vi "ADIS16470 Reset.vi"(8 "error in (no error)":errorcluster, 10 "Reset?":bool, 11 "ADIS16470DevRef":T1) -> (0 "error out":errorcluster, 3 "ADIS16470DevRef":T1)   [LabVIEW 2018]
uses:
  Typedef/ADIS16470 Device Reference.ctl
  Typedef/ADIS16470 Hardware Configuration.ctl
  <vilib>/Rock Robotics/WPI/SPI/WPI_SPIMode.ctl
  <vilib>/Rock Robotics/SystemInterfaces/DIO/FPGA_DIOChannel.ctl
  <vilib>/Rock Robotics/SystemInterfaces/spilib/spi_bus.ctl
  Typedef/ADIS16470 Data.ctl
  Typedef/ADIS16470 Status.ctl
  Typedef/ADIS16470 Process.ctl
  Typedef/ADIS16470 Command Type.ctl
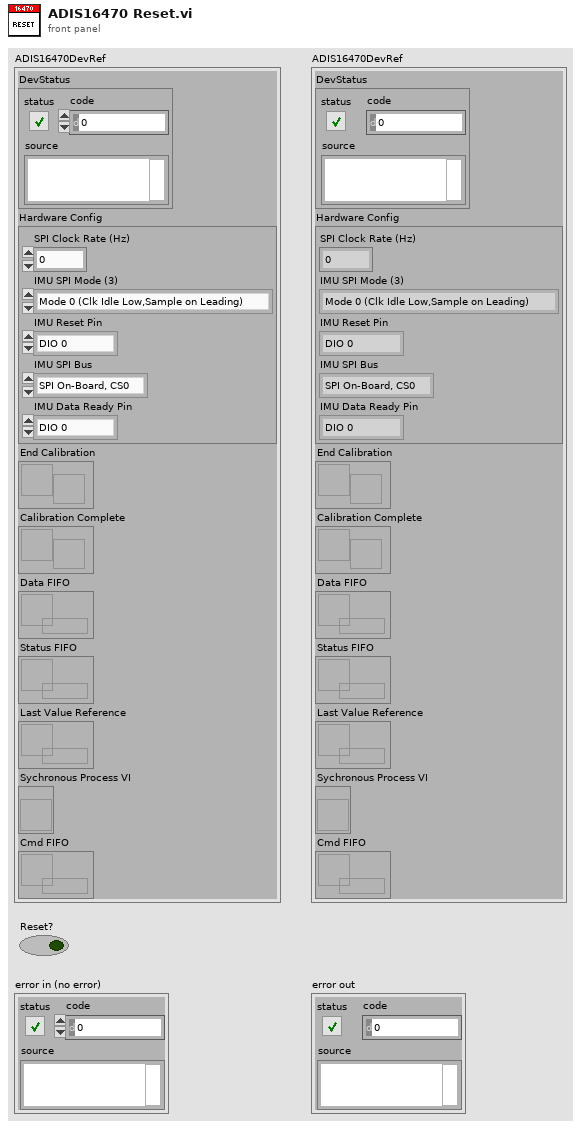
[diagram p1: front panel]
types:
  T1 = typedef "ADIS16470 Device Reference.ctl" = cluster{"DevStatus":errorcluster, "Hardware Config":T2, "End Calibration":refnum<notifier>, "Calibration Complete":refnum<notifier>, "Data FIFO":refnum<k33>, "Status FIFO":refnum<k33>, "Last Value Reference":refnum<data-value>, "Sychronous Process VI":T6, "Cmd FIFO":refnum<k33>}
  T2 = typedef "ADIS16470 Hardware Configuration.ctl" = cluster{"SPI Clock Rate (Hz)":dbl, "IMU SPI Mode (3)":T3, "IMU Reset Pin":T4, "IMU SPI Bus":T5, "IMU Data Ready Pin":T4}
  T3 = typedef "WPI_SPIMode.ctl" = enum16{"Mode 0 (Clk Idle Low,Sample on Leading)", "Mode 1 (Clk Idle Low,Sample on Trailing)", "Mode 2 (Clk Idle High,Sample on Leading)", "Mode 3 (Clk Idle High,Sample on Trailing)"}
  T4 = typedef "FPGA_DIOChannel.ctl" = enum8{"DIO 0", "DIO 1", "DIO 2", "DIO 3", "DIO 4", "DIO 5", "DIO 6", "DIO 7", "DIO 8", "DIO 9", "DIO MXP 0", "DIO MXP 1", "DIO MXP 2", "DIO MXP 3", "DIO MXP 4", "DIO MXP 5", "DIO MXP 6", "DIO MXP 7", "DIO MXP 8", "DIO MXP 9", "DIO MXP 10", "DIO MXP 11", "DIO MXP 12", "DIO MXP 13", "DIO MXP 14", "DIO MXP 15", "SPI Port CS1", "SPI Port CS2", "SPI Port CS3", "SPI Port MISO", "SPI Port MOSI", "Invalid"}
  T5 = typedef "spi_bus.ctl" = enum16{"SPI On-Board, CS0", "SPI On-Board, CS1", "SPI On-Board, CS2", "SPI On-Board, CS3", "SPI MXP", "Invalid"}
  T6 = typedef "ADIS16470 Process.ctl" = refnum<vi>
  T7 = typedef "ADIS16470 Command Type.ctl" = enum16{"None", "Reset"}
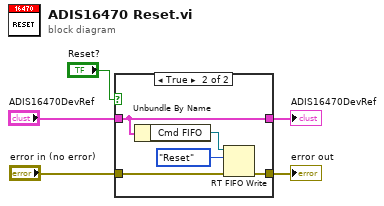
[diagram p0: block diagram]
diagram:
  n1 = case shown="True" "Reset?" {
    tunnel: "ADIS16470DevRef" -> [w6 w10]
    tunnel: "error in (no error)" -> [w7 w12]
    tunnel: [w7 w11] -> w4
    tunnel: [w6 w10] -> w5
    frame False {
    }
    frame True {
      n2 = Unbundle By Name(w10) -> ("Cmd FIFO"=w9:refnum<k33>)
      n3 = RT FIFO Write(0:w9, 1:ADIS16470_Command_Type."Reset" ("element"), 3:w12) -> (11:w11:errorcluster)  [unwired: 2 in, 3 out]
    }
  }
  "ADIS16470DevRef" <- w5
  "error out" <- w4
